vi "TCP-Connection.vi"(8 "error in":errorcluster, 10 "Mode":enum16{"TCP-Lost", "Write", "Read"}(ring)=enum."Write", 11 "connection info":T1) -> (0 "error out":errorcluster, 2 "NewVal?":bool, 3 "connection info Out":T1)   [LabVIEW 2016]
uses:
  <vilib>/NI/STM/TCP/TCP Connection Info.ctl
  <vilib>/NI/STM/SubVIs/MetaDataElement.ctl
  <vilib>/ErrorRing/Error Ring.xnode
  <vilib>/NI/STM/NI STM.lvlib
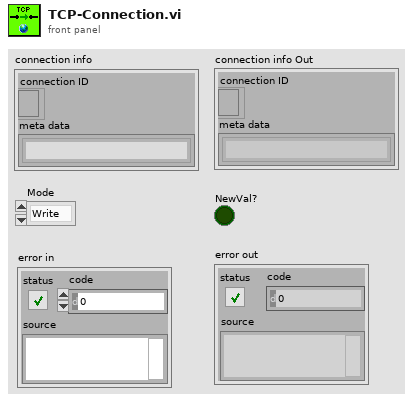
[diagram p1: front panel]
types:
  T1 = typedef "NI STM.lvlib/TCP Connection Info.ctl" = cluster{"connection ID":refnum<k5>, "meta data":T2[]}
  T2 = typedef "NI STM.lvlib/MetaDataElement.ctl" = string
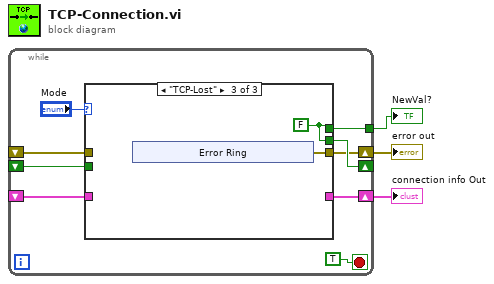
[diagram p0: block diagram]
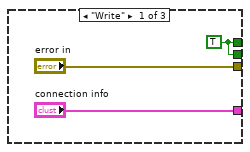
[diagram p2: hidden frame]
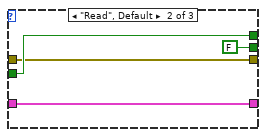
[diagram p3: hidden frame]
diagram:
  n1 = while {
    shift-right: [w11] -> _
    shift-left: _ -> [w10]
    shift-right: [w8] -> w3
    shift-left: _ -> [w7]
    tunnel: [w6] -> w2
    shift-right: [w5] -> w1
    shift-left: _ -> [w4]
    stop <- TRUE stop-if-true
    n2 = case shown="\"TCP-Lost\"" "Mode" {
      tunnel: [w14 FALSE w20] -> w11
      tunnel: w10 -> [_ w17 _]
      tunnel: ["connection info" w19 _] -> w8
      tunnel: w7 -> [_ w19 _]
      tunnel: [w14 w17 w20] -> w6
      tunnel: w4 -> [_ w16 _]
      tunnel: ["error in" w16 w21] -> w5
      frame "Write" {
        w14 = TRUE
      }
      frame "Read", Default {
      }
      frame "TCP-Lost" {
        w20 = FALSE
        n3 = xnode "Error Ring"() -> ("error out"=w21:errorcluster)
      }
    }
  }
  "NewVal?" <- w2
  "error out" <- w1
  "connection info Out" <- w3
